vi "KE622x -- Get Arm Output Mode.vi"(0 "Resource In":refnum<visa-resource-name>, 1 "Check For SCPI Errors? (T)":bool=TRUE, 11 "error in (no error)":errorcluster) -> (4 "Resource Out (dupl)":refnum<visa-resource-name>, 8 "Arm Output Mode":T1, 15 "error out":errorcluster)   [LabVIEW 2018, in "Keithley 622x.lvlib"]
uses:
  Keithley 622x.lvlib
  Typedefs/KE622x -- Arm Output Mode.ctl
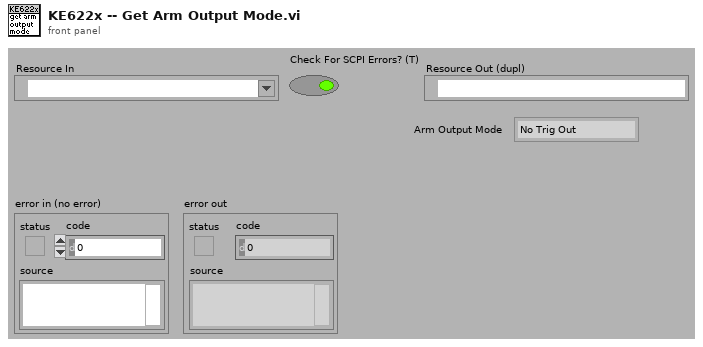
[diagram p1: front panel]
types:
  T1 = typedef "Keithley 622x.lvlib/KE622x -- Arm Output Mode.ctl" = enum16{"No Trig Out", "Trig Out On Enter Arm", "Trig Out On Exit Arm"}
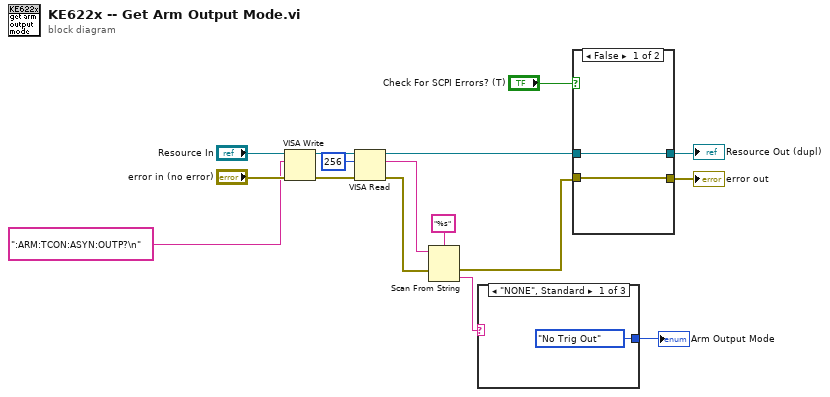
[diagram p0: block diagram]
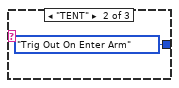
[diagram p2: hidden frame]
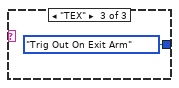
[diagram p3: hidden frame]
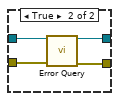
[diagram p4: hidden frame]
diagram:
  n1 = VISA Write(VISA resource name="Resource In", write buffer=":ARM:TCON:ASYN:OUTP?\n" ("format string"), error in (no error)="error in (no error)") -> (VISA resource name out=w10:refnum<visa-resource-name>, error out=w9:errorcluster)  [unwired: 1 out]
  n2 = VISA Read(VISA resource name=w10, byte count=u32 256, error in (no error)=w9) -> (VISA resource name out=w3:refnum<visa-resource-name>, read buffer=w5:string, error out=w7:errorcluster)  [unwired: 1 out]
  n3 = Scan From String(format string="%s", input string=w5, error in=w7) -> (error out=w4:errorcluster, output 1=w2:string)  [unwired: 2 in, 2 out]
  n4 = case shown="\"NONE\", Standard" w2 {
    tunnel: [KE622x_--_Arm_Output_Mode."No Trig Out" ("Arm Output Mode") KE622x_--_Arm_Output_Mode."Trig Out On Enter Arm" ("Arm Output Mode") KE622x_--_Arm_Output_Mode."Trig Out On Exit Arm" ("Arm Output Mode")] -> w1
    frame "NONE", Default {
    }
    frame "TENT" {
    }
    frame "TEX" {
    }
  }
  "Arm Output Mode" <- w1
  n5 = case shown="False" "Check For SCPI Errors? (T)" {
    tunnel: w3 -> [w21 w25]
    tunnel: w4 -> [w20 w24]
    tunnel: [w20 w23] -> w12
    tunnel: [w21 w22] -> w13
    frame False {
    }
    frame True {
      n6 = call "Error Query.vi"("VISA Resource In"=w25, "error in (no error)"=w24) -> ("VISA Resource Out (dupl)"=w22:refnum<visa-resource-name>, "error out"=w23:errorcluster)  [unwired: 10 in, 2 out]
    }
  }
  "Resource Out (dupl)" <- w13
  "error out" <- w12
